vi "DB Get Test Preset ID.vi"(5 "Queue in":refnum<queue>, 7 "DB":refnum<queue>, 8 "error in (no error)":errorcluster, 11 "Setting in":T1 {"PS Measure Plan" items=["Pretreatment settings (PS)", "Linear Sweep Voltammetry (LSV)", "Differential Pulse Voltammetry (DPV)", "Cyclic Voltammetry (CV)", "Chronoamperometry (CA)", "Chronopotentiometry (CP)", "El Imp Spectroscopy (EIS)"]; "System Preset"."Test Configuration"."SP List" format="%#.1g"}) -> (0 "error out":errorcluster, 3 "Setting out":T1 {"PS Measure Plan" items=["Pretreatment settings (PS)", "Linear Sweep Voltammetry (LSV)", "Differential Pulse Voltammetry (DPV)", "Cyclic Voltammetry (CV)", "Chronoamperometry (CA)", "Chronopotentiometry (CP)", "El Imp Spectroscopy (EIS)"]; "System Preset"."Test Configuration"."SP List" format="%#.1g"})   [LabVIEW 2020, in "Settings.lvlib"]
uses:
  Settings.lvlib
  support/Message Queue/Message Queue.lvlib
  support/PCT FGV CMD.ctl
  support/Message Queue/Message Cluster.ctl
  Test Driver/System Preset.ctl
  Test Driver/Test Type.ctl
  Test Driver/Test Driver.lvlib
  Test Driver/Test Driver Configuration.ctl
panel:
  # "X"
  # "Y"
  # "Cycles"
  # "Point Delay"
  # "Up"
  # "Down"
  # "Z Axes"
  # "#C"
  # "In"
  # "Out"
  # "Cleaning [sec]"
  # "X"
  # "Y"
  # "Cycles"
  # "Point Delay"
  # "Up"
  # "Down"
  # "Z Axes"
  # "#C"
  # "In"
  # "Out"
  # "Cleaning [sec]"
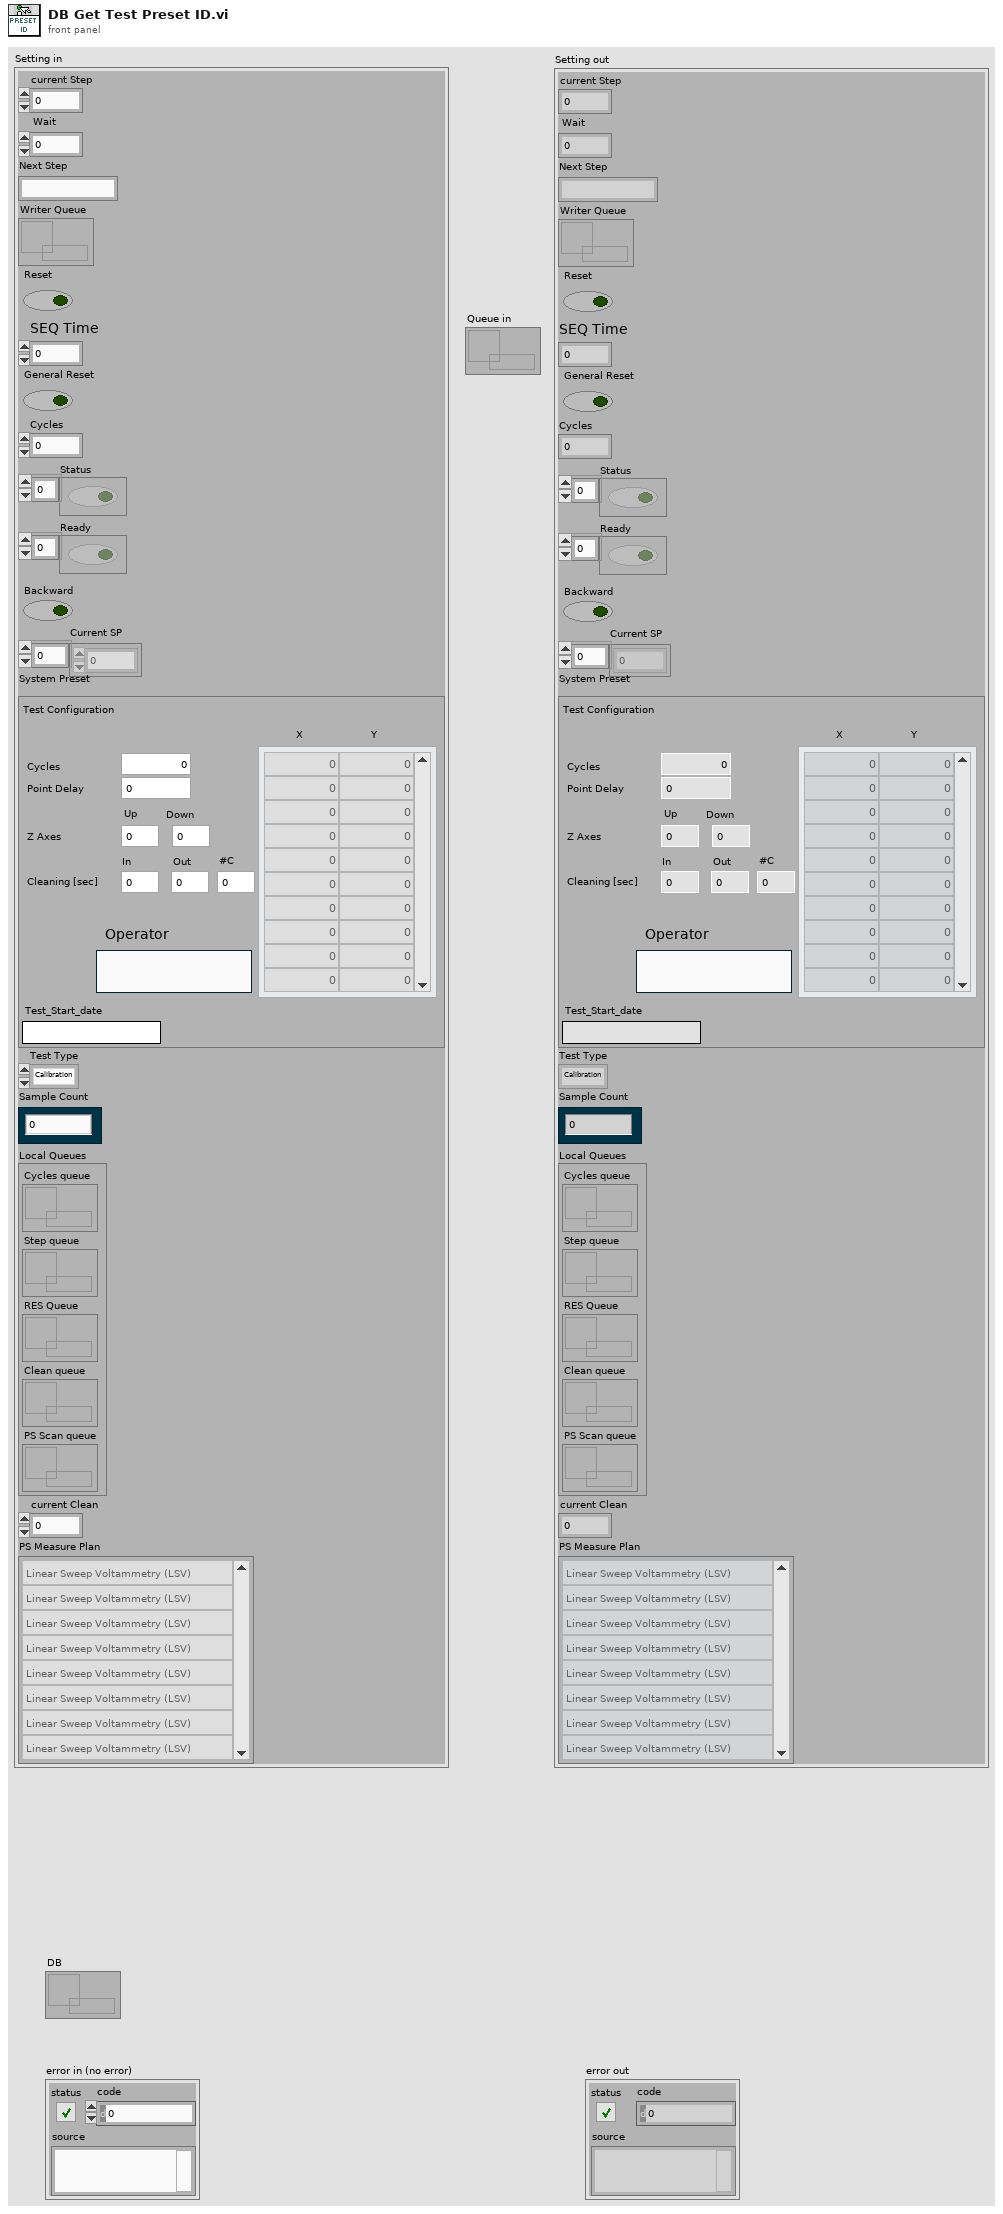
[diagram p1: front panel]
types:
  T1 = typedef "Test Driver.lvlib/Test Driver Configuration.ctl" = cluster{"current Step":i32, "Wait":dbl, "Next Step":string, "Writer Queue":refnum<queue>, "Reset":bool, "SEQ Time":i32, "General Reset":bool, "Cycles":i32, "Status":bool[], "Ready":bool[], "Backward":bool, "Current SP":dbl[], "System Preset":T2, "Test Type":T3, "Sample Count":i32, "Local Queues":cluster{"Cycles queue":refnum<queue>, "Step queue":refnum<queue>, "RES Queue":refnum<queue>, "Clean queue":refnum<queue>, "PS Scan queue":refnum<queue>}, "current Clean":i32, "PS Measure Plan":u16[]}
  T2 = typedef "System Preset.ctl" = cluster{"Test Configuration":cluster{"Cycles":i32, "Z Up":dbl, "SP List":dbl[][], "Operator":string, "Point Delay":i32, "Z Up 2":dbl, "Cleaning In":dbl, "Cleaning Out":dbl, "Cleaning Cycles":i32}, "Test_Start_date":string}
  T3 = typedef "Test Driver.lvlib/Test Type.ctl" = enum16{"Calibration", "Test"}
  T4 = cluster{"Type CMD":string, "Mode CMD":string, "Main CMD":string}
  T5 = typedef "PCT FGV CMD.ctl" = enum16{"INIT", "GET", "SET"}
  T6 = cluster{"Wire Type":string, "Adhesive Type":string, "Solder Type":string, "Z Up":dbl}
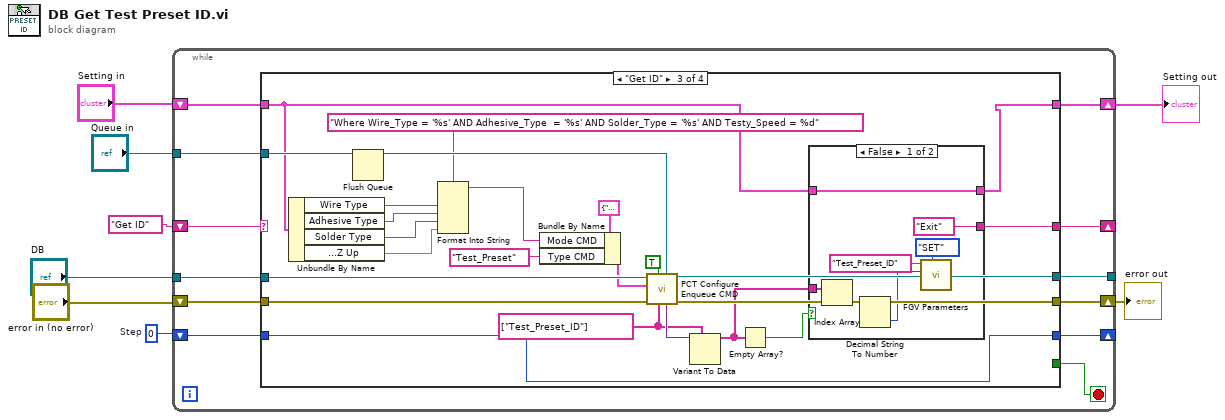
[diagram p0: block diagram]
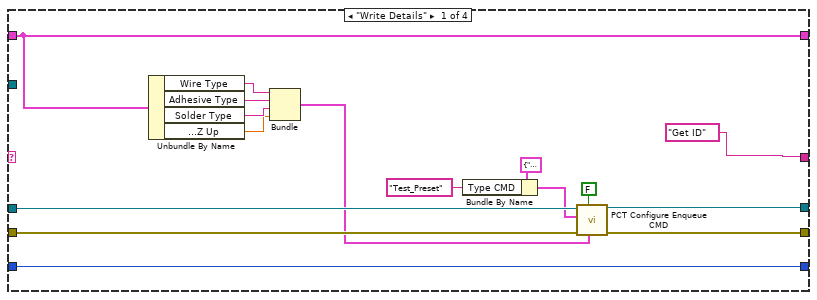
[diagram p2: hidden frame]
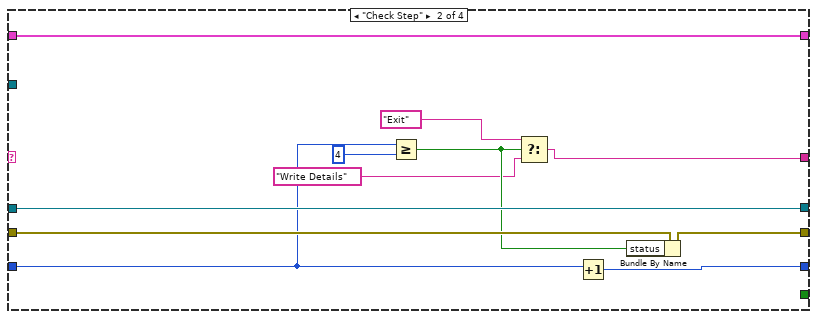
[diagram p3: hidden frame]
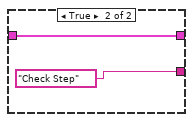
[diagram p4: hidden frame]
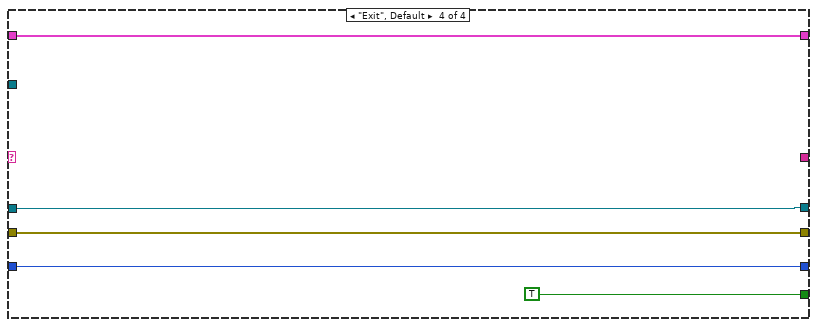
[diagram p5: hidden frame]
diagram:
  w5 = 0  # Step
  n1 = while {
    shift-right: [w15] -> _
    shift-left: "Get ID" ("CMD") -> [w20]
    shift-right: [w18] -> w6
    shift-left: "error in (no error)" -> [w19]
    tunnel: "DB" -> [w17]
    tunnel: [w16] -> _
    tunnel: "Queue in" -> [w14]
    shift-right: [w12] -> w3
    shift-left: "Setting in" -> [w13]
    shift-right: [w9] -> _
    shift-left: w5 -> [w10]
    stop <- w11 stop-if-true
    n2 = case shown="\"Get ID\"" w20 {
      tunnel: w19 -> [w36 w45 w71 w84]
      tunnel: [w35 w39 w70 w84] -> w18
      tunnel: w17 -> [w34 w46 w69 w85]
      tunnel: [w33 w46 w68 w85] -> w16
      tunnel: ["Get ID" ("CMD") w41 w57 _] -> w15
      tunnel: w14 -> [_ _ w65 _]
      tunnel: w13 -> [w28 w40 w56 w81]
      tunnel: [w28 w40 w55 w81] -> w12
      tunnel: [_ _ _ TRUE] -> w11
      tunnel: w10 -> [w29 w44 w53 w82]
      tunnel: [w29 w47 w53 w82] -> w9
      frame "Write Details" {
        n3 = Unbundle By Name(w28) -> ("Wire Type"=w26:string, "Adhesive Type"=w25:string, "Solder Type"=w24:string, "System Preset.Test Configuration.Z Up"=w23:dbl)
        n4 = Bundle("Wire Type"=w26, "Adhesive Type"=w25, "Solder Type"=w24, "Z Up"=w23) -> (w22:T6)  [unwired: 1 in]
        n5 = Bundle By Name(cluster=T4 {"Type CMD"="System_Configuration", "Mode CMD"="Swept SA", "Main CMD"="Insert Data"} ("CMD"), "Type CMD"="Test_Preset") -> (w32:T4)
        n6 = call "PCT Configure Enqueue CMD.vi"("Parameter Data"=w22, "Read"=FALSE, "error in (no error)"=w36, "CMD"=w32, "CMD Queue in"=w34) -> ("error out"=w35:errorcluster, "CMD Queue out"=w33:refnum<queue>)  [unwired: 4 in, 1 out]
      }
      frame "Check Step" {
        n7 = Greater Or Equal?(x=w44, y=4) -> (x >= y?=w38:bool)
        n8 = Select(t="Exit" ("CMD"), s=w38, f="Write Details" ("CMD")) -> (s? t:f=w41:string)
        n9 = Increment(x=w44) -> (x+1=w47:i32)
        n10 = Bundle By Name(cluster=w45, "status"=w38) -> (w39:errorcluster)
      }
      frame "Get ID" {
        w60 = string[] ["Test_Preset_ID"]
        n11 = Unbundle By Name(w56) -> ("Wire Type"=w48:string, "Adhesive Type"=w51:string, "Solder Type"=w50:string, "System Preset.Test Configuration.Z Up"=w49:dbl)
        n12 = Flush Queue(queue=w65) -> (queue out=w64:refnum<queue>)  [unwired: 1 in, 2 out]
        n13 = Format Into String(format string="Where Wire_Type = '%s' AND Adhesive_Type  = '%s' AND Solder_Type = '%s' AND Testy_Speed = %d", w48, w51, w50, w49) -> (resulting string=w62:string)  [unwired: 2 in, 1 out]
        n14 = Bundle By Name(cluster=T4 {"Type CMD"="System_Configuration", "Mode CMD"="Swept SA", "Main CMD"="Get Data"} ("CMD"), "Mode CMD"=w62, "Type CMD"="Test_Preset" ("CMD")) -> (w67:T4)
        n15 = call "PCT Configure Enqueue CMD.vi"("Response Queue"=w64, "Parameter Data"=w60, "Read"=TRUE, "error in (no error)"=w71, "CMD"=w67, "CMD Queue in"=w69) -> ("error out"=w70:errorcluster, "CMD Queue out"=w68:refnum<queue>, "Message Data"=w61:variant)  [unwired: 3 in]
        n16 = Variant To Data(type=w60, Variant=w61) -> (data=w58:string[])  [unwired: 1 in, 1 out]
        n17 = Empty Array?(array=w58) -> (empty?=w59:bool)
        n18 = case shown="False" w59 {
          tunnel: w58 -> [w78 _]
          tunnel: ["Exit" ("CMD") "Check Step" ("CMD")] -> w57
          tunnel: [w76 w80] -> w55
          tunnel: w56 -> [w76 w80]
          frame False {
            n19 = Index Array(array=w78) -> (element=w77:string)  [unwired: 1 in]
            n20 = Decimal String To Number(string=w77) -> (number=w73:i32)  [unwired: 2 in, 1 out]
            n21 = call "FGV Parameters.vi"("CMD"=PCT_FGV_CMD."SET", "input"=w73, "Key"="Test_Preset_ID") -> ()  [unwired: 6 in, 3 out]
          }
          frame True {
          }
        }
      }
      frame "Exit", Default {
      }
    }
  }
  "error out" <- w6
  "Setting out" <- w3
